vi "QCA Save Channels.vi"() -> (0 "Error":bool)   [LabVIEW 2010]
uses:
  QCA Global.vi
  TPS Global.vi
  <vilib>/Utility/config.llb/NI_LVConfig.lvlib
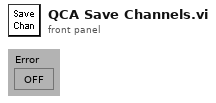
[diagram p1: front panel]
types:
  T1 = cluster{"Name":string, "Type":enum16{"I32", "DBL", "STR"}, "Changeable":bool}[]
  T2 = typedef "NI_LVConfig.lvlib/Config Data RefNum.ctl" = refnum<k1>
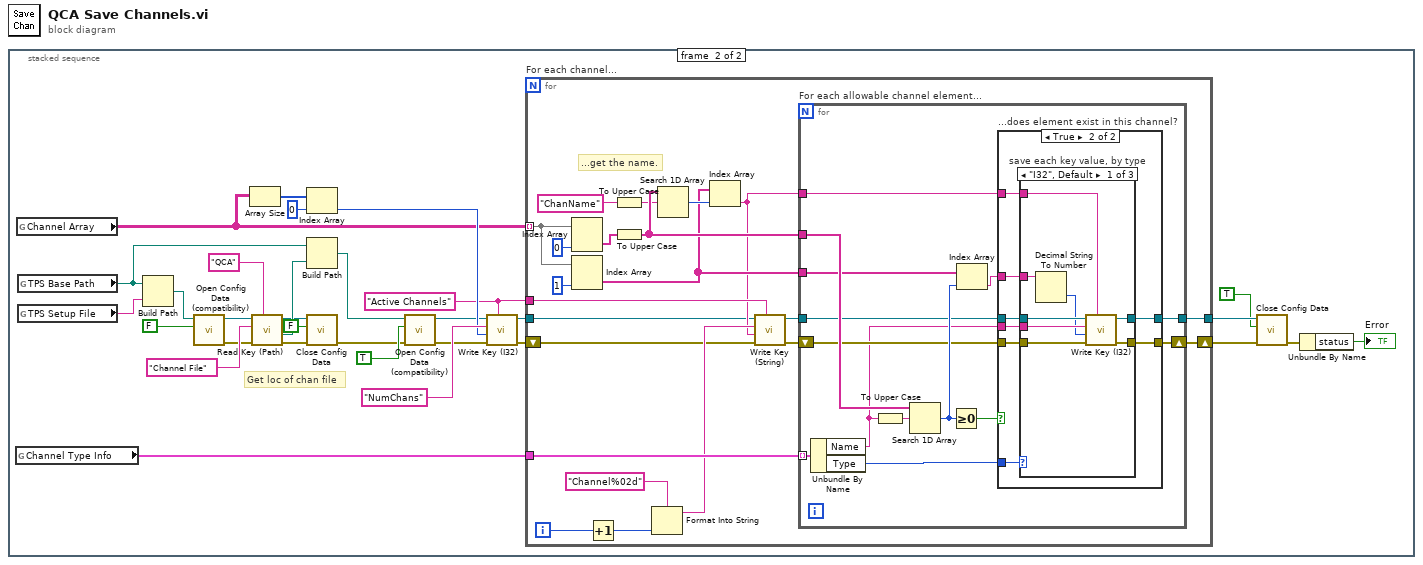
[diagram p0: block diagram]
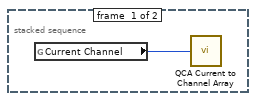
[diagram p2: hidden frame]
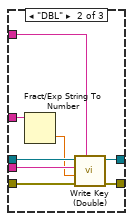
[diagram p4: hidden frame]
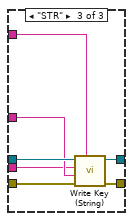
[diagram p5: hidden frame]
diagram:
  n1 = stacked-sequence {
    frame #0 {
      n2 = global read "QCA Global.vi" "Current Channel"() -> (w1:i32)
      n3 = call "QCA Current to Channel Array.vi"("Channel Number"=w1) -> ()
    }
    frame #1 {
      w6 = "Active Channels" ("section")
      # "Get loc of chan file"
      n4 = global read "QCA Global.vi" "Channel Type Info"() -> (w13:T1)
      n5 = global read "QCA Global.vi" "Channel Array"() -> (w16:string[][][])
      n6 = global read "TPS Global.vi" "TPS Base Path"() -> (w29:path)
      n7 = global read "TPS Global.vi" "TPS Setup File"() -> (w7:string)
      n8 = Build Path(base path=w29, name or relative path=w7) -> (appended path=w21:path)
      n9 = call <vilib>:"Open Config Data (compatibility).vi"("create file if necessary (T)"=FALSE ("create file if necessary? (T)"), "configuration file path"=w21) -> ("error out"=w23:errorcluster, "refnum"=w24:T2)  [unwired: 7 in, 1 out]
      n10 = Array Size(array=w16) -> (size(s)=w32:i32[])
      n11 = call <vilib>:"Read Key (Path).vi"("section"="QCA", "error in (no error)"=w23, "key"="Channel File", "refnum"=w24) -> ("error out"=w26:errorcluster, "value"=w30:path, "refnum out"=w25:T2)  [unwired: 4 in, 1 out]
      n12 = Index Array(array=w32, index=0 ("Index")) -> (element=w19:i32)
      n13 = Build Path(base path=w29, name or relative path=w30) -> (appended path=w3:path)
      n14 = call <vilib>:"Close Config Data.vi"("error in (no error)"=w26, "write file if changed (T)"=FALSE, "refnum"=w25) -> ("error out"=w4:errorcluster)  [unwired: 7 in, 1 out]
      n15 = call <vilib>:"Open Config Data (compatibility).vi"("error in (no error)"=w4, "create file if necessary (T)"=TRUE ("create file if necessary? (T)"), "configuration file path"=w3) -> ("error out"=w18:errorcluster, "refnum"=w17:T2)  [unwired: 6 in, 1 out]
      n16 = call <vilib>:"Write Key (I32).vi"("section"=w6, "error in (no error)"=w18, "value"=w19, "key"="NumChans", "refnum"=w17) -> ("error out"=w15:errorcluster, "refnum out"=w14:T2)  [unwired: 4 in, 1 out]
      n17 = for "For each channel..." {
        tunnel: w16 -> [w54] mode=indexing
        shift-right: [w34] -> w12
        shift-left: w15 -> [w38]
        tunnel: w14 -> [w39]
        tunnel: w13 -> [w48]
        tunnel: [w33] -> w11
        tunnel: w6 -> [w44]
        i -> [w41]
        # "...get the name."
        n18 = Index Array(array=w54, index (col)=0 ("Index")) -> (element=w53:string[])  [unwired: 1 in]
        n19 = Index Array(array=w54, index (col)=1 ("Index")) -> (element=w49:string[])  [unwired: 1 in]
        n20 = Increment(x=w41) -> (x+1=w35:i32)
        n21 = To Upper Case(1:"ChanName" ("element")) -> (0:w47:string)
        n22 = To Upper Case(1:w53) -> (0:w50:string[])
        n23 = Format Into String(format string="Channel%02d" ("Format String"), w35) -> (resulting string=w42:string)  [unwired: 2 in, 1 out]
        n24 = Search 1D Array(1D array=w50, element=w47) -> (index of element=w51:i32)  [unwired: 1 in]
        n25 = Index Array(array=w49, index=w51) -> (element=w40:string)
        n26 = call <vilib>:"Write Key (String).vi"("section"=w44, "error in (no error)"=w38, "value"=w40, "key"=w42, "refnum"=w39) -> ("error out"=w37:errorcluster, "refnum out"=w36:T2)  [unwired: 4 in, 1 out]
        n27 = for "For each allowable channel element..." {
          tunnel: w40 -> [w68]
          tunnel: w50 -> [w66]
          tunnel: w49 -> [w64]
          tunnel: w48 -> [w67] mode=indexing
          shift-right: [w59] -> w34
          shift-left: w37 -> [w60]
          tunnel: w36 -> [w58]
          tunnel: [w55] -> w33
          n28 = Unbundle By Name(w67) -> ("Name"=w57:string, "Type"=w61:enum16{"I32", "DBL", "STR"})
          n29 = To Upper Case(1:w57) -> (0:w56:string)
          n30 = Search 1D Array(1D array=w66, element=w56) -> (index of element=w63:i32)  [unwired: 1 in]
          n31 = Greater Or Equal To 0?(x=w63) -> (x >= 0?=w62:bool)
          n32 = Index Array(array=w64, index=w63) -> (element=w65:string)
          n33 = case "...does element exist in this channel?" shown="True" w62 {
            tunnel: w68 -> [_ w78]
            tunnel: w65 -> [_ w77]
            tunnel: w61 -> [_ w76]
            tunnel: w60 -> [w70 w75]
            tunnel: [w70 w74] -> w59
            tunnel: w58 -> [w69 w73]
            tunnel: w57 -> [_ w72]
            tunnel: [w69 w71] -> w55
            frame False {
              # "do nothing."
            }
            frame True {
              n34 = case "save each key value, by type" shown="\"I32\", Default" w76 {
                tunnel: w73 -> [w86 w94 w101]
                tunnel: w75 -> [w85 w93 w100]
                tunnel: [w84 w92 w99] -> w74
                tunnel: [w83 w91 w98] -> w71
                tunnel: w78 -> [w82 w90 w97]
                tunnel: w77 -> [w80 w88 w96]
                tunnel: w72 -> [w81 w89 w95]
                frame "I32", Default {
                  n35 = Decimal String To Number(string=w80) -> (number=w79:i32)  [unwired: 2 in, 1 out]
                  n36 = call <vilib>:"Write Key (I32).vi"("section"=w82, "error in (no error)"=w85, "value"=w79, "key"=w81, "refnum"=w86) -> ("error out"=w84:errorcluster, "refnum out"=w83:T2)  [unwired: 4 in, 1 out]
                }
                frame "DBL" {
                  n37 = Fract/Exp String To Number(string=w88) -> (number=w87:dbl)  [unwired: 3 in, 1 out]
                  n38 = call <vilib>:"Write Key (Double).vi"("section"=w90, "error in (no error)"=w93, "value"=w87, "key"=w89, "refnum"=w94) -> ("error out"=w92:errorcluster, "refnum out"=w91:T2)  [unwired: 4 in, 1 out]
                }
                frame "STR" {
                  n39 = call <vilib>:"Write Key (String).vi"("section"=w97, "error in (no error)"=w100, "value"=w96, "key"=w95, "refnum"=w101) -> ("error out"=w99:errorcluster, "refnum out"=w98:T2)  [unwired: 4 in, 1 out]
                }
              }
            }
          }
        }
      }
      n40 = call <vilib>:"Close Config Data.vi"("error in (no error)"=w12, "write file if changed (T)"=TRUE ("write configuration file? (F)"), "refnum"=w11) -> ("error out"=w8:errorcluster)  [unwired: 7 in, 1 out]
      n41 = Unbundle By Name(w8) -> ("status"=→"Error":bool)
    }
  }
